vi "DownItem__slk_tc.vi"(0 "tree control in":refnum<class "TreeControl.lvclass">, 5 "indent tag (current tag)":string, 11 "error in (no error)":errorcluster) -> (4 "tree control out":refnum<class "TreeControl.lvclass">, 15 "error out":errorcluster)   [LabVIEW 2020, in "TreeControl.lvclass"]
doc: "Moves the input tag item lower."
uses:
  Library/TreeControl.lvclass
  Library/TreeControl.lvclass/TreeControl.ctl
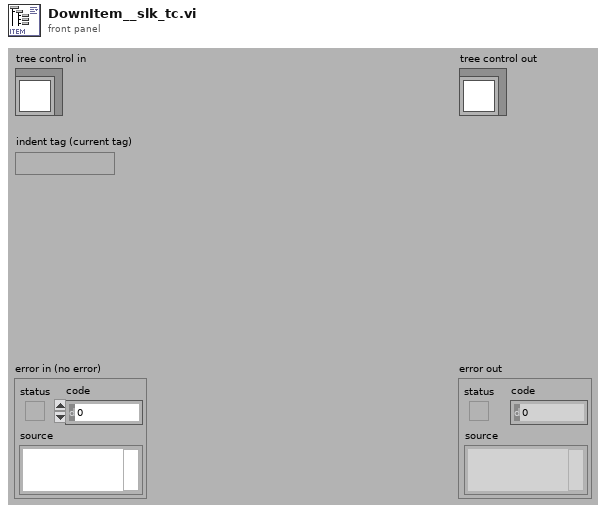
[diagram p1: front panel]
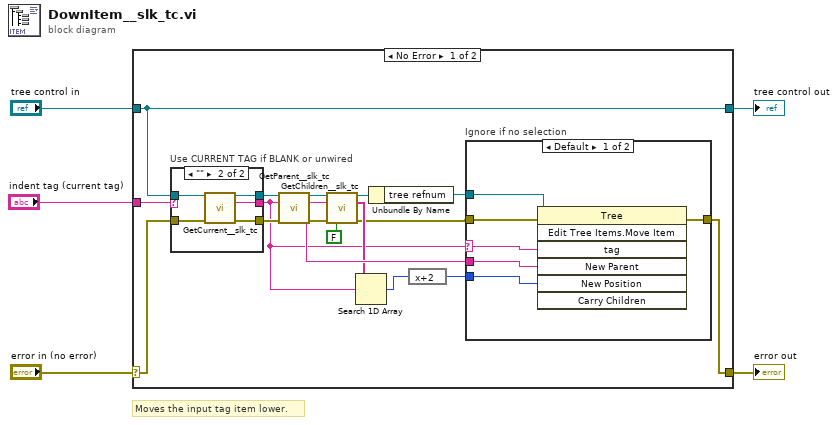
[diagram p0: block diagram]
diagram:
  # "Moves the input tag item lower."
  n1 = case shown="No Error" "error in (no error)" {
    selector: "error in (no error)" -> [w10 w39]
    tunnel: [w9 w39] -> w4
    tunnel: [w22 w38] -> w2
    tunnel: "tree control in" -> [w22 w38]
    tunnel: "indent tag (current tag)" -> [w8 _]
    frame No Error {
      n2 = case "Use CURRENT TAG if BLANK or unwired" shown="\"\"" w8 {
        selector: w8 -> [w32 _]
        tunnel: [w32 w37] -> w13
        tunnel: w22 -> [w30 w36]
        tunnel: w10 -> [w31 w35]
        tunnel: [w31 w34] -> w19
        tunnel: [w30 w33] -> w20
        frame Default {
        }
        frame "" {
          n3 = call "GetCurrent__slk_tc.vi"("tree control in"=w36, "error in (no error)"=w35) -> ("tree control out"=w33:refnum<class "TreeControl.lvclass">, "current tag"=w37:string, "error out"=w34:errorcluster)  [unwired: 1 in, 10 out]
        }
      }
      n4 = call "GetParent__slk_tc.vi"("tree control in"=w20, "child tag (\"\")"=w13, "error in (no error)"=w19) -> ("tree control out"=w18:refnum<class "TreeControl.lvclass">, "parent tag"=w16:string, "error out"=w17:errorcluster)  [unwired: 10 out]
      n5 = call "GetChildren__slk_tc.vi"("tree control in"=w18, "parent tag (\"\")"=w16, "error in (no error)"=w17, "use current (T)"=FALSE) -> ("tree control out"=w14:refnum<class "TreeControl.lvclass">, "children tags"=w15:string[], "error out"=w11:errorcluster)  [unwired: 9 out]
      n6 = Search 1D Array(1D array=w15, element=w13) -> (index of element=w12:i32)  [unwired: 1 out]
      n7 = Unbundle By Name(w14) -> ("tree refnum"=w21:refnum<vi>)
      n8 = expression code="x+2"(w12) -> (w6:i32)
      n9 = case "Ignore if no selection" shown="Default" w13 {
        selector: w13 -> [w27 _]
        tunnel: w21 -> [w26 _]
        tunnel: w11 -> [w28 w29]
        tunnel: [w25 w29] -> w9
        tunnel: w16 -> [w24 _]
        tunnel: w6 -> [w23 _]
        frame Default {
          n10 = invoke class="Tree" method="Edit Tree Items.Move Item"(reference=w26, error in=w28, "tag"=w27, "New Parent"=w24, "New Position"=w23) -> (error out=w25:errorcluster)  [unwired: 2 in, 6 out]
        }
        frame "" {
        }
      }
    }
    frame Error {
    }
  }
  "error out" <- w4
  "tree control out" <- w2
